vi "Initialize.vi"(8 "error in (no error)":errorcluster, 11 "Device in":refnum<class "Device.lvclass">) -> (0 "error out":errorcluster, 3 "Device out":refnum<class "Device.lvclass">)   [LabVIEW 2020, in "Device.lvlib" / "Device.lvclass"]
uses:
  Device.lvclass
  DeviceStatus.ctl
  Device.lvclass/Device.ctl
  Device.lvlib
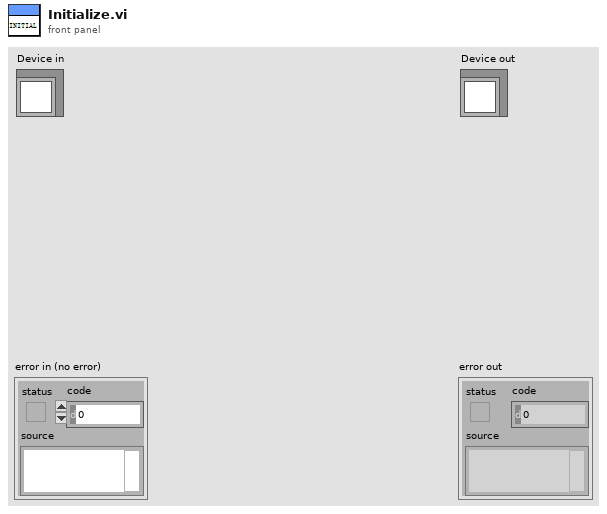
[diagram p1: front panel]
types:
  T1 = typedef "Device.lvlib/DeviceStatus.ctl" = i32
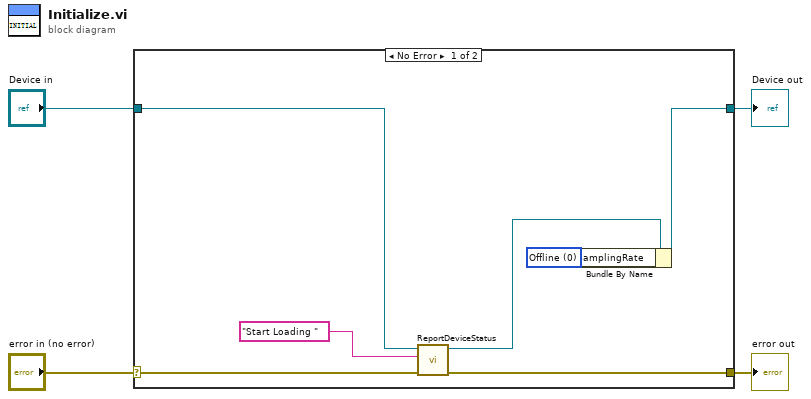
[diagram p0: block diagram]
diagram:
  n1 = case shown="No Error" "error in (no error)" {
    selector: "error in (no error)" -> [w11 w13]
    tunnel: [w10 w13] -> w3
    tunnel: [w6 w12] -> w1
    tunnel: "Device in" -> [w9 w12]
    frame No Error {
      w5 = T1 0 items=["Offline", "Idle", "Busy"] ("Status")
      n2 = call-dynamic "ReportDeviceStatus.vi"("error in (no error)"=w11, "Status"="Start Loading ", "Device in"=w9) -> ("error out"=w10:errorcluster, "Device out"=w8:refnum<class "Device.lvclass">)  [unwired: 7 in]
      n3 = Bundle By Name(cluster=w8, "SamplingRate"=w5) -> (w6:refnum<class "Device.lvclass">)
    }
    frame Error {
    }
  }
  "error out" <- w3
  "Device out" <- w1
